vi "ClassPanel.vi"(8 "error in (no error)":errorcluster caption="entrée d'erreur (pas d'erreur)", 11 "Tools.lvclass":refnum<class "Tools.lvclass">) -> (0 "error out":errorcluster caption="sortie d'erreur", 3 "Tools.lvclass Out":refnum<class "Tools.lvclass">)   [LabVIEW 2019, in "Tools.lvclass"]
uses:
  Tools.lvclass
  C:/Programmes Labview/LabScanV1A/DevicesClass/BaseDevice/BaseDevice.lvclass
  BaseDevice/Accessor/GetClassEvent.vi
panel:
  in  "Acq":bool
  in  "MainProgQ":refnum<queue>
  in  "MainProgQEvent":refnum<user-event>
  in  "Stop":bool
  out "TempsRest":dbl caption="Temps Restant" format="%<%H:%M:%S%1u>t"
  in  "MiseAJour":bool
  in  "Intervalle":dbl=60.0 caption="Acq. Interval" min=0.1 step=0.1 format="%#.1f"
  out "Init Program":bool
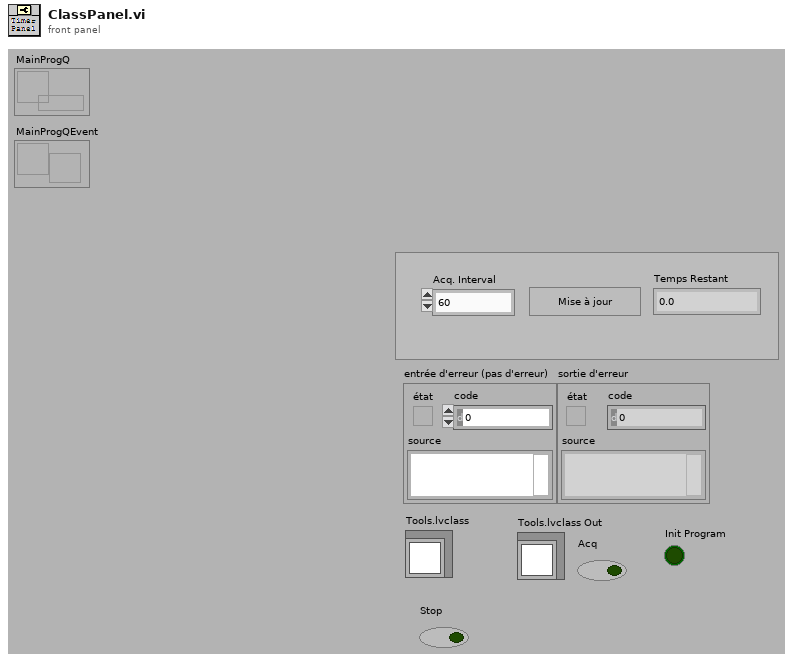
[diagram p1: front panel]
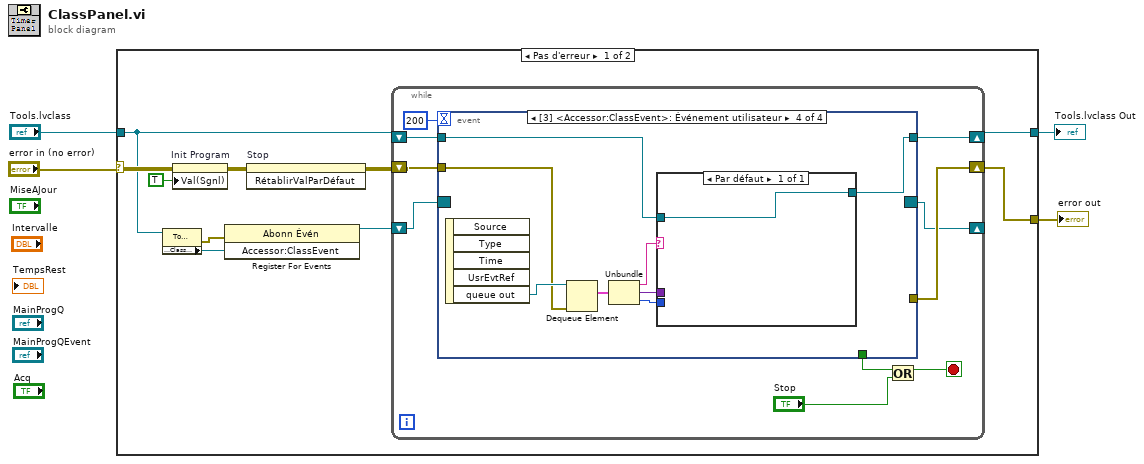
[diagram p0: block diagram]
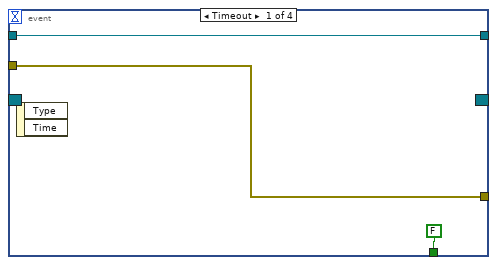
[diagram p2: hidden frame]
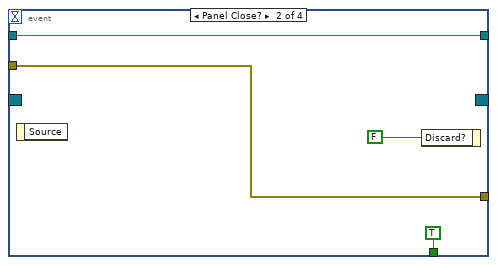
[diagram p3: hidden frame]
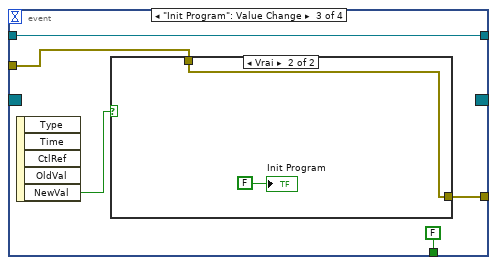
[diagram p4: hidden frame]
diagram:
  n1 = case shown="Pas d'erreur" "error in (no error)" {
    selector: "error in (no error)" -> [w11 w50]
    tunnel: [w14 w50] -> w3
    tunnel: "Tools.lvclass" -> [w6 w49]
    tunnel: [w12 w49] -> w1
    frame No Error {
      n2 = property class="Tools.lvclass"(reference=w6) -> (error out=w7:errorcluster, "Accessor:ClassEvent"=w8:refnum<user-event>)  [unwired: 1 in, 1 out]
      n3 = property on="Init Program" class="Bool (strict)"(error in=w11, "Val(Sgnl)"=TRUE ("Valeur (Signalisation)")) -> (error out=w10:errorcluster)  [unwired: 1 in, 1 out]
      n4 = register-events(error in=w7, w8) -> (reference out=w5:refnum<event-registration>)  [unwired: 1 in, 1 out]
      n5 = invoke on="Stop" class="Bool (strict)" method="RétablirValParDéfaut"(error in=w10) -> (error out=w9:errorcluster)  [unwired: 2 in, 2 out]
      n6 = while {
        shift-right: [w22] -> w14
        shift-left: w9 -> [w23]
        shift-right: [w19] -> w12
        shift-left: w6 -> [w21]
        shift-right: [w15] -> _
        shift-left: w5 -> [w16]
        stop <- w18 stop-if-true
        n7 = event shown="[3] <Accessor:ClassEvent>: Événement utilisateur" {
          selector: w16 -> [_ _ _ _]
          dyn-events: [_ _ _ _] -> w15
          timeout: 200 -> [_ _ _ _]
          tunnel: w23 -> [w25 w29 w35 w45]
          tunnel: [w25 w29 w34 _] -> w22
          tunnel: w21 -> [w26 w28 w33 w40]
          tunnel: [FALSE TRUE FALSE _] -> w20
          tunnel: [w26 w28 w33 w41] -> w19
          event Timeout {
            n8 = event-data() -> ()  [unwired: 1 in, 2 out]
          }
          event Panel Close? {
            n9 = event-data() -> ()  [unwired: 1 in, 1 out]
            n10 = event-data("Discard?"=FALSE ("Rejeter ?")) -> ()  [unwired: 1 in, 1 out]
          }
          event "Init Program": Value Change {
            n11 = event-data() -> ("NewVal"=w36:bool)  [unwired: 1 in, 4 out]
            n12 = case shown="Vrai" w36 {
              tunnel: w35 -> [w37 w38]
              tunnel: [w37 w38] -> w34
              frame False {
              }
              frame True {
                "Init Program" <- FALSE
              }
            }
          }
          event User Event {
            n13 = event-data() -> ("queue out"=w46:refnum<queue>)  [unwired: 1 in, 4 out]
            n14 = Dequeue Element(queue=w46, error in (no error)=w45) -> (element=w47:cluster{"Message":string, "Data":variant, i32})  [unwired: 1 in, 3 out]
            n15 = Unbundle(w47) -> ("Message"=w44:string, "Data"=w43:variant, w42:i32)
            n16 = case shown="Par défaut" w44 {
              tunnel: w43 -> [_]
              tunnel: w42 -> [_]
              tunnel: [w48] -> w41
              tunnel: w40 -> [w48]
              frame Par défaut {
              }
            }
          }
        }
        n17 = Or(x=w20, y="Stop") -> (x .or. y?=w18:bool)
      }
    }
    frame Error {
    }
  }
  "error out" <- w3
  "Tools.lvclass Out" <- w1
